vi "InitDeviceManager.vi"(6 "If monitor: show panel?":bool=TRUE, 7 "Monitor ICL":bool=TRUE, 8 "error in (no error)":errorcluster, 9 "start ICL on local host?":bool=TRUE, 10 "WS Server Port":string="25010", 11 "WS Server IP":string="ws://127.0.0.1") -> (0 "error out":errorcluster, 3 "device manager":refnum<class "DeviceManager.lvclass">)   [LabVIEW 2023, in "DeviceManager.lvclass"]
uses:
  DeviceManager.lvclass
  DeviceManager.lvclass/DeviceManager.ctl
  32339246-19d0-4101-aa43-29dff1db1305.vi
  Communicator/Communicator.lvclass
panel:
  # "Connector Pane"
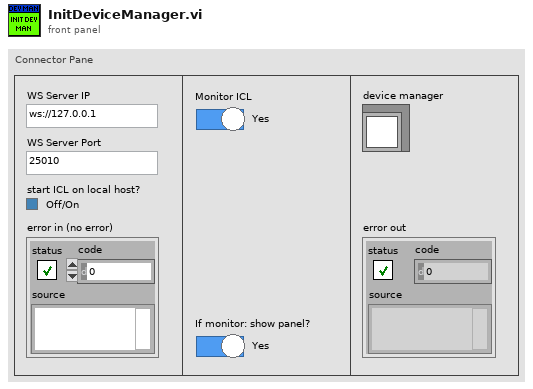
[diagram p1: front panel]
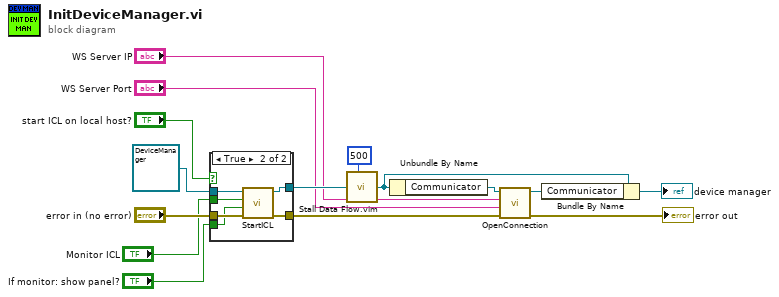
[diagram p0: block diagram]
diagram:
  n1 = case shown="True" "start ICL on local host?" {
    tunnel: refnum<class "DeviceManager.lvclass"> refnum ("DeviceManager.lvclass") -> [w17 w23]
    tunnel: [w17 w22] -> w13
    tunnel: "error in (no error)" -> [w16 w21]
    tunnel: [w16 w20] -> w8
    tunnel: "Monitor ICL" -> [_ w19]
    tunnel: "If monitor: show panel?" -> [_ w18]
    frame False {
    }
    frame True {
      n2 = call-dynamic "StartICL.vi"("error in (no error)"=w21, "If monitor: show panel?"=w18, "Monitor ICL"=w19, "DeviceManager in"=w23) -> ("error out"=w20:errorcluster, "DeviceManager out"=w22:refnum<class "DeviceManager.lvclass">)  [unwired: 6 in]
    }
  }
  n3 = call "Stall Data Flow.vim"("value in"=w13, "milliseconds to wait"=u32 500) -> ("value out"=w7:refnum<class "DeviceManager.lvclass">)  [unwired: 1 out]
  n4 = Unbundle By Name(w7) -> ("Communicator"=w12:refnum<class "Communicator.lvclass">)
  n5 = call-dynamic "OpenConnection.vi"("error in (no error)"=w8, "WS Server Port"="WS Server Port", "WS Server IP"="WS Server IP", "Communicator in"=w12) -> ("error out"=→"error out":errorcluster, "Communicator out"=w6:refnum<class "Communicator.lvclass">)  [unwired: 5 in, 1 out]
  n6 = Bundle By Name(cluster=w7, "Communicator"=w6) -> (→"device manager":refnum<class "DeviceManager.lvclass">)
